vi "StringList.Get Items.vi"(8 "error in (no error)":errorcluster, 11 "StringList in":refnum<class "StringList.lvclass">) -> (0 "error out":errorcluster, 2 "Items Out":string[](array[string]), 3 "StringList out":refnum<class "StringList.lvclass">)   [LabVIEW 2024, in "StringList.lvclass"]
uses:
  StringList.lvclass
  StringList.lvclass/StringList.ctl
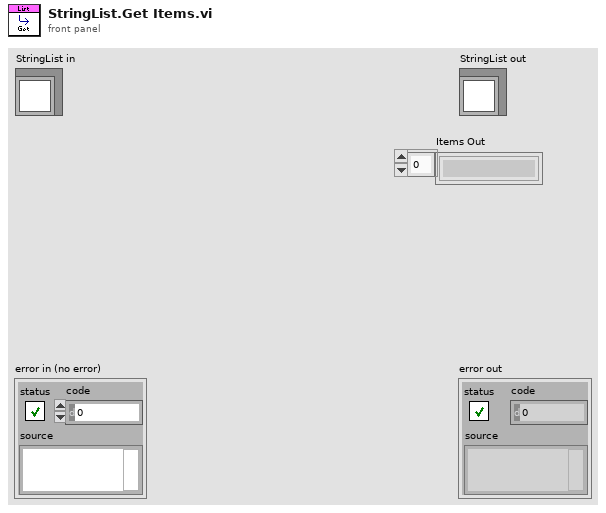
[diagram p1: front panel]
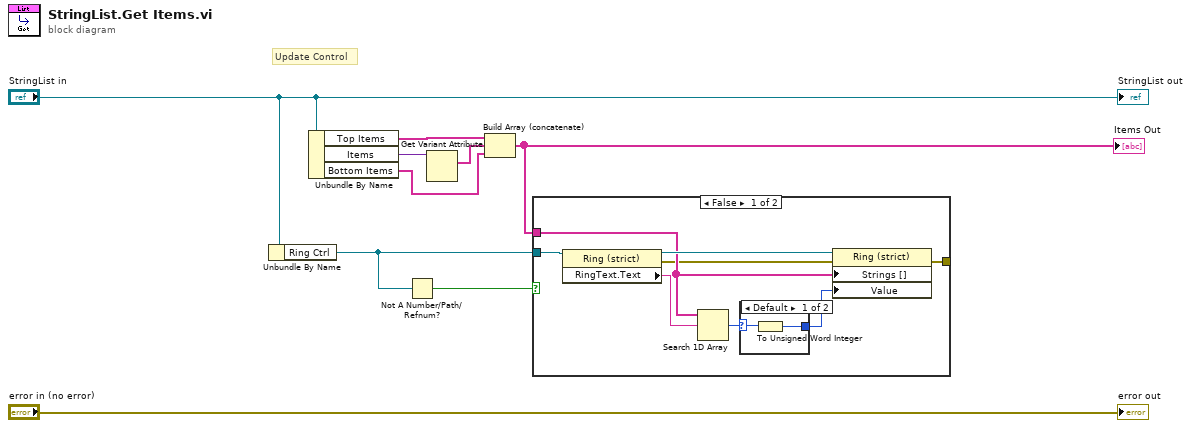
[diagram p0: block diagram]
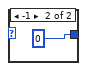
[diagram p2: hidden frame]
diagram:
  # "Update Control"
  n1 = Unbundle By Name("StringList in") -> ("Ring Ctrl"=w7:refnum<vi>)
  n2 = Unbundle By Name("StringList in") -> ("Top Items"=w6:string[], "Items"=w4:variant, "Bottom Items"=w5:string[])
  n3 = Not A Number/Path/Refnum?(number/path/refnum=w7) -> (NaN/Path/Refnum?=w2:bool)
  n4 = Get Variant Attribute(Variant=w4) -> (names=w3:string[])  [unwired: 3 in, 3 out]
  n5 = Build Array (concatenate)(w6, w3, w5) -> (w8:string[])
  "Items Out" <- w8
  n6 = case shown="False" w2 {
    tunnel: w7 -> [w17 _]
    tunnel: w8 -> [w15 _]
    tunnel: [w11 _] -> _
    frame False {
      n7 = property class="Ring (strict)"(reference=w17) -> (reference out=w16:refnum<vi>, error out=w10:errorcluster, "RingText.Text"=w14:string)  [unwired: 1 in]
      n8 = Search 1D Array(1D array=w15, element=w14) -> (index of element=w13:i32)  [unwired: 1 in]
      n9 = case shown="Default" w13 {
        selector: w13 -> [w19 _]
        tunnel: [w18 u16 0 ("Value")] -> w12
        frame Default {
          n10 = To Unsigned Word Integer(number=w19) -> (unsigned 16bit integer=w18:u16)
        }
        frame -1 {
        }
      }
      n11 = property class="Ring (strict)"(reference=w16, error in=w10, "Strings []"=w15, "Value"=w12) -> (error out=w11:errorcluster)  [unwired: 1 out]
    }
    frame True {
    }
  }
  "error out" <- "error in (no error)"
  "StringList out" <- "StringList in"
